vi "DefaultFromINI.vi"(8 "error in (no error)":errorcluster, 11 "AcPwrBase":refnum<class "AcPwrBase.lvclass">) -> (0 "error out":errorcluster, 3 "AcPwrBase":refnum<class "AcPwrBase.lvclass">)   [LabVIEW 2018, in "AcPwrPlugins.lvlib" / "AcPwrBase.lvclass"]
doc: "This VI loads the instruments' configuration previously stored on file."
uses:
  AcPwrBase.lvclass
  C:/Program Files (x86)/National Instruments/LabVIEW 2018/user.lib/NIST/BaseClasses/BasePlugin_class/BasePlugin.lvclass
  TypeDefs/BaseConfig.ctl
  TypeDefs/Phase.ctl
  TypeDefs/BaseMeasurements.ctl
  ChromaAcLoadClass/TypeDefs/MeasurementType.ctl
  <userlib>/NIST/BaseClasses/BasePlugin_class/BasePlugin.lvclass/BasePlugin.ctl
  AcPwrBase.lvclass/AcPwrBase.ctl
  <userlib>/NIST/BaseClasses/BasePlugin_class/Accessors/Read PluginIniFilePath.vi
  <userlib>/NIST/BaseClasses/BasePlugin_class/Accessors/Write PluginIniFilePath.vi
  Accessors/Write BaseConfig.vi
  <vilib>/Utility/config.llb/NI_LVConfig.lvlib
  ChromaAcLoadClass/ChromaAcLoad.lvclass
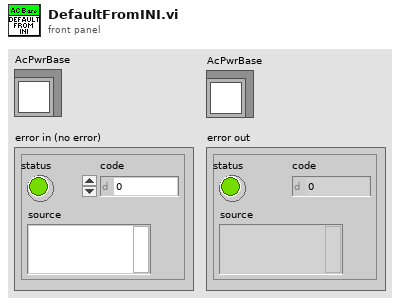
[diagram p1: front panel]
types:
  T1 = typedef "AcPwrPlugins.lvlib/AcPwrBase.lvclass/BaseMeasurements.ctl" = cluster{"Handle":string, "Name":string, "Enabled":bool, "Measurement Value":dbl, "btnMeasFetch":bool, "Chroma Hold Peak Current Measurement":bool, "Chroma Measurement Type":T2, "Chroma Protection Status String":string, "NHRDC Fetch Method":i32, "NHRDC Fetch Time (s)":sgl, "NHRDC Measurement Type":i32, "NHRGridSim Measurement Type ":enum16{"Average Current", "Max Current", "Min Current", "Average Voltage", "Max Voltage", "Min Voltage", "Average True Power", "Max True Power", "Min True Power", "Average Apparent Power", "Max Apparent Power", "Min Apparent Power", "Power Factor", "Crest Factor"}, "NHRGridSim Phase ":i32, "PPS Measurement Type ":enum16{"Voltage RMS L-N", "Voltage RMS L-L", "Frequency", "Current RMS", "Current Peak", "Crest Factor", "Power Factor", "Power VA", "Real Power"}, "PPS Channel Name":enum16{"A", "B", "C"}}[]
  T2 = typedef "AcPwrPlugins.lvlib/ChromaAcLoad.lvclass/MeasurementType.ctl" = enum16{"Voltage (Vrms or V)", "Current (Arms or A)", "Power (W)", "Peak Voltage (V)", "Peak Current (A)", "Peak Power (W)", "Frequency (Hz)", "Resistance (Ohms)", "Voltage Overshoot (V)", "Positive Peak Current (A)", "Voltage Undershoot (V)", "Negative Peak Current (A)", "Apparent Power (VA)", "Reacitive Power (VAR)", "Voltage THD", "Power Factor", "Current's Crest Factor"}
  T3 = typedef "AcPwrPlugins.lvlib/AcPwrBase.lvclass/BaseConfig.ctl" = cluster{"Frequency":dbl, "FrequencyRange":dbl[], "Phases":T4[], "Name":string, "PluginConfigVariant":variant, "PluginMeasVariant":variant}
  T4 = typedef "AcPwrPlugins.lvlib/AcPwrBase.lvclass/Phase.ctl" = cluster{"Name":string, "Enabled":bool, "VoltageLevel":dbl, "Handle":string, "VoltageRange":dbl[], "Connected":bool, "CurrentLimit":dbl, "Waveform":string}
  T5 = typedef "NI_LVConfig.lvlib/Config Data RefNum.ctl" = refnum<k1>
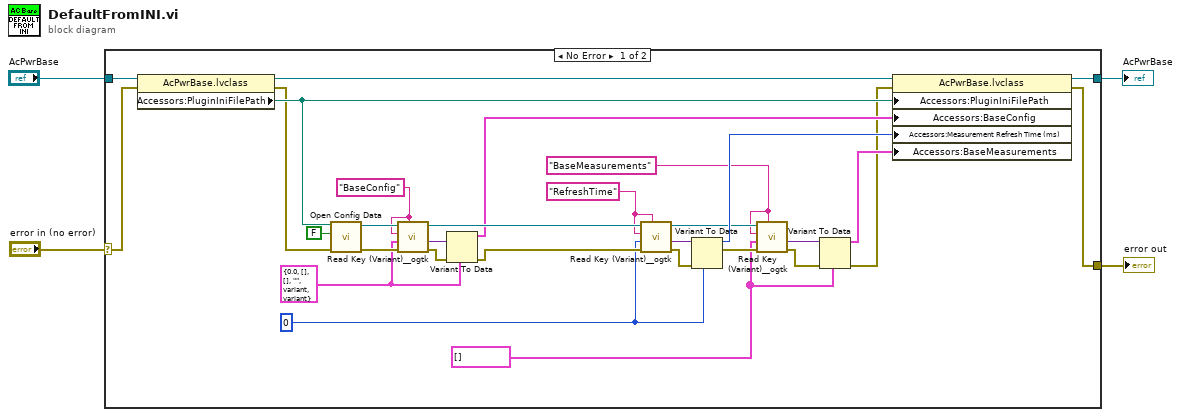
[diagram p0: block diagram]
diagram:
  n1 = case shown="No Error" "error in (no error)" {
    selector: "error in (no error)" -> [w10 w36]
    tunnel: "AcPwrBase" -> [w26 w35]
    tunnel: [w27 w35] -> w3
    tunnel: [w9 w36] -> w2
    frame No Error {
      w12 = T1 [] ("BaseMeasurements")
      w11 = "BaseMeasurements" ("section")
      w19 = u32 0
      w13 = "RefreshTime" ("section")
      w5 = T3 {"Frequency"=0.0, "FrequencyRange"=[], "Phases"=[], "Name"="", "PluginConfigVariant"=variant, "PluginMeasVariant"=variant(cluster{"MeasName":string, "Modules":cluster{"Handle":string, "Connected":bool, "Clear Device (F)":bool, "btnIdQuery":bool, "btnReset":bool, "Program #":cluster{"Phase B (Degrees)":i32, "Waveform A (1: Sine)":i32, "Voltage Level (Va)":dbl, "Program Number (0)":i32, "Voltage Level (Vb) ":dbl, "Form (3: Three)":u16, "Coupling  (0: Direct)":u16, "Frequency (45Hz)":dbl, "Current Limit (40A)":dbl, "Phase C (Degrees)":i32, "Voltage Level (Vc)":dbl, "Waveform B (1: Sine)":i32, "Waveform C (1: Sine)":i32}[], "Impedance Parameters (off, 0.00)":cluster{"State":bool, "Impedance":dbl}, "Transient Execution (F)":bool, "OutputEnabled":bool, "Source Range":cluster{"Frequency Minimum (45 Hz)":dbl, "Frequency Maximum (1200 Hz)":dbl, "Voltage Maximum (V)":dbl, "Voltage Minimum (V)":dbl, "Range Control (0: Auto)":u16, "Initial Voltage (0V)":u16, "Frequency Range (600Hz)":u16}, "Port Type":enum16{"GPIB", "Serial"}}[]} {"MeasName"="", "Modules"=[]})} ("BaseConfig")
      w6 = "BaseConfig" ("section (optional)")
      n2 = property class="AcPwrBase.lvclass"(reference=w26, error in=w10) -> (reference out=w25:refnum<class "AcPwrBase.lvclass">, error out=w7:errorcluster, "Accessors:PluginIniFilePath"=w24:path)
      n3 = call <vilib>:"Open Config Data.vi"("error in (no error)"=w7, "create file if necessary (T)"=FALSE, "configuration file path"=w24) -> ("error out"=w31:errorcluster, "refnum"=w32:T5)  [unwired: 6 in, 1 out]
      n4 = call <userlib>:"Read Key (Variant)__ogtk.vi"("section"=w6, "error in (no error)"=w31, "type"=w5, "key (optional)"=w6, "refnum"=w32) -> ("error out"=w30:errorcluster, "key-value"=w34:variant, "refnum out"=w29:T5)  [unwired: 3 in, 1 out]
      n5 = Variant To Data(error in=w30, type=w5, Variant=w34) -> (data=w23:T3, error out=w28:errorcluster)
      n6 = call <userlib>:"Read Key (Variant)__ogtk.vi"("section"=w13, "error in (no error)"=w28, "type"=w19, "key (optional)"=w13, "refnum"=w29) -> ("error out"=w21:errorcluster, "key-value"=w22:variant, "refnum out"=w17:T5)  [unwired: 3 in, 1 out]
      n7 = Variant To Data(error in=w21, type=w19, Variant=w22) -> (data=w20:u32, error out=w18:errorcluster)
      n8 = call <userlib>:"Read Key (Variant)__ogtk.vi"("section"=w11, "error in (no error)"=w18, "type"=w12, "key (optional)"=w11, "refnum"=w17) -> ("error out"=w16:errorcluster, "key-value"=w15:variant)  [unwired: 3 in, 2 out]
      n9 = Variant To Data(error in=w16, type=w12, Variant=w15) -> (data=w14:T1, error out=w8:errorcluster)
      n10 = property class="AcPwrBase.lvclass"(reference=w25, error in=w8, "Accessors:PluginIniFilePath"=w24, "Accessors:BaseConfig"=w23, "Accessors:Measurement Refresh Time (ms)"=w20, "Accessors:BaseMeasurements"=w14) -> (reference out=w27:refnum<class "AcPwrBase.lvclass">, error out=w9:errorcluster)
    }
    frame Error {
    }
  }
  "error out" <- w2
  "AcPwrBase" <- w3
